vi "video_global.vi"() -> ()   [LabVIEW 2015]
uses:
  <vilib>/LVH/AR Drone Toolkit/Type Defs/AR Drone Resource.ctl
  <vilib>/LVH/AR Drone Toolkit/AR Drone.lvlib
panel:
  out "NR poza":dbl=1.0
  out "Snap photo":bool
  out "Video Stream":picture
  out "AR Drone Resource":T1={"UDP Control Connection"=refnum, "UDP NavData Connection"=refnum, "UDP Video Connection (Drone 1.0)"=refnum, "TCP Video Connection (Drone 2.0)"=refnum, "TCP Control Port Connection"=refnum, "Drone IP address"="192.168.1.1", "Drone Command Port"=5556, "Drone NavData Port"=5554, "Drone Vid Stream Port"=5555, "Drone TCP Control Port"=5559, "Home IP address"="192.168.1.2", "Home Command Port"=56828, "Home NavData Port"=56829, "Home Vid Stream Port"=56830, "Drone Version"=0, "Drone Index"=0, "Command Sequence"=1}
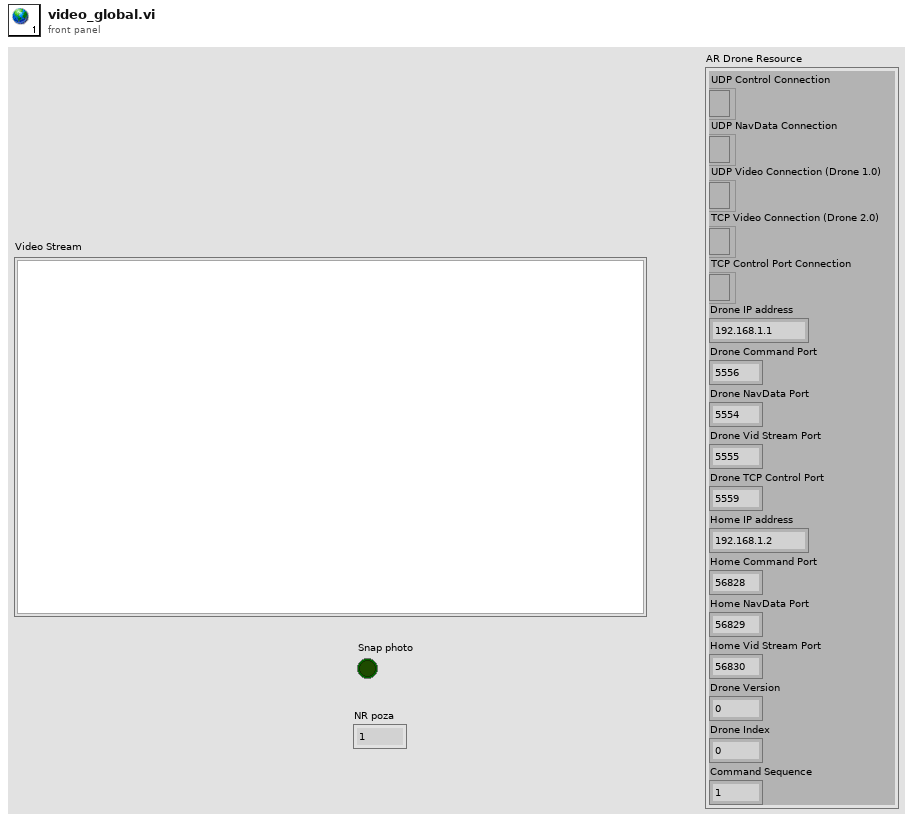
[diagram p1: front panel]
types:
  T1 = typedef "AR Drone.lvlib/AR Drone Resource.ctl" = cluster{"UDP Control Connection":refnum<k16>, "UDP NavData Connection":refnum<k16>, "UDP Video Connection (Drone 1.0)":refnum<k16>, "TCP Video Connection (Drone 2.0)":refnum<k5>, "TCP Control Port Connection":refnum<k5>, "Drone IP address":string, "Drone Command Port":u16, "Drone NavData Port":u16, "Drone Vid Stream Port":u16, "Drone TCP Control Port":u16, "Home IP address":string, "Home Command Port":u16, "Home NavData Port":u16, "Home Vid Stream Port":u16, "Drone Version":i32, "Drone Index":i32, "Command Sequence":i32}
diagram:
